vi "Unregister and Destroy Sessions.vi"(8 "error in (no error)":errorcluster) -> (0 "error out":errorcluster)   [LabVIEW 2020, in "NI-DCPower Source DC Voltage.lvlib"]
uses:
  NI-DCPower Source DC Voltage.lvlib
  <vilib>/MeasurementLink/MeasurementLink Discovery Client/RPC Messages/ni_measurementlink_discovery_v1_ResolveServiceRequest.ctl
  <vilib>/MeasurementLink/MeasurementLink Session Management Client/RPC Messages/ni_measurementlink_sessionmanagement_v1_ReserveAllRegisteredSessionsRequest.ctl
  <vilib>/MeasurementLink/MeasurementLink Session Management Client/MeasurementLink Session Management Client.lvlib
  <vilib>/MeasurementLink/MeasurementLink Discovery Client/MeasurementLink Discovery Client.lvlib
  <vilib>/MeasurementLink/MeasurementLink Measurement Server/MeasurementLink Measurement Server.lvlib
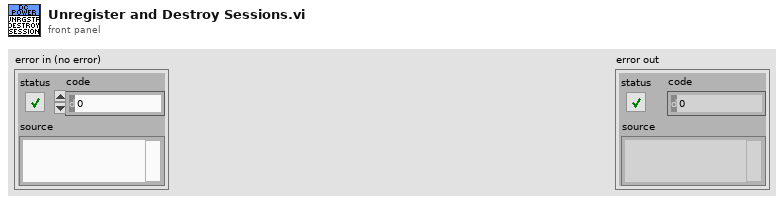
[diagram p1: front panel]
types:
  T1 = typedef "MeasurementLink Session Management Client.lvlib/ni_measurementlink_sessionmanagement_v1_ReserveAllRegisteredSessionsRequest.ctl" = cluster{"timeout_in_milliseconds":i32, "instrument_type_id":string}
  T2 = typedef "MeasurementLink Discovery Client.lvlib/ni_measurementlink_discovery_v1_ResolveServiceRequest.ctl" = cluster{"provided_interface":string, "service_class":string}
  T3 = typedef "grpc-lvsupport-release.lvlib/grpcId.ctl" = u64
  T4 = typedef "MeasurementLink Discovery Client.lvlib/ni_measurementlink_discovery_v1_ServiceLocation.ctl" = cluster{"location":string, "insecure_port":string, "ssl_authenticated_port":string}
  T5 = typedef "MeasurementLink Session Management Client.lvlib/ni_measurementlink_sessionmanagement_v1_ReserveAllRegisteredSessionsResponse.ctl" = cluster{"sessions":T6[]}
  T6 = typedef "MeasurementLink Session Management Client.lvlib/ni_measurementlink_sessionmanagement_v1_SessionInformation.ctl" = cluster{"session":T7, "resource_name":string, "channel_list":string, "instrument_type_id":string, "session_exists":bool, "channel_mappings":T8[]}
  T7 = typedef "MeasurementLink Session Management Client.lvlib/nidevice_grpc_Session.ctl" = cluster{"name":string}
  T8 = typedef "MeasurementLink Session Management Client.lvlib/ni_measurementlink_sessionmanagement_v1_ChannelMapping.ctl" = cluster{"pin_or_relay_name":string, "site":i32, "channel":string}
  T9 = cluster{"session Name":string, "address (localhost)":string, "port (31763)":i32}
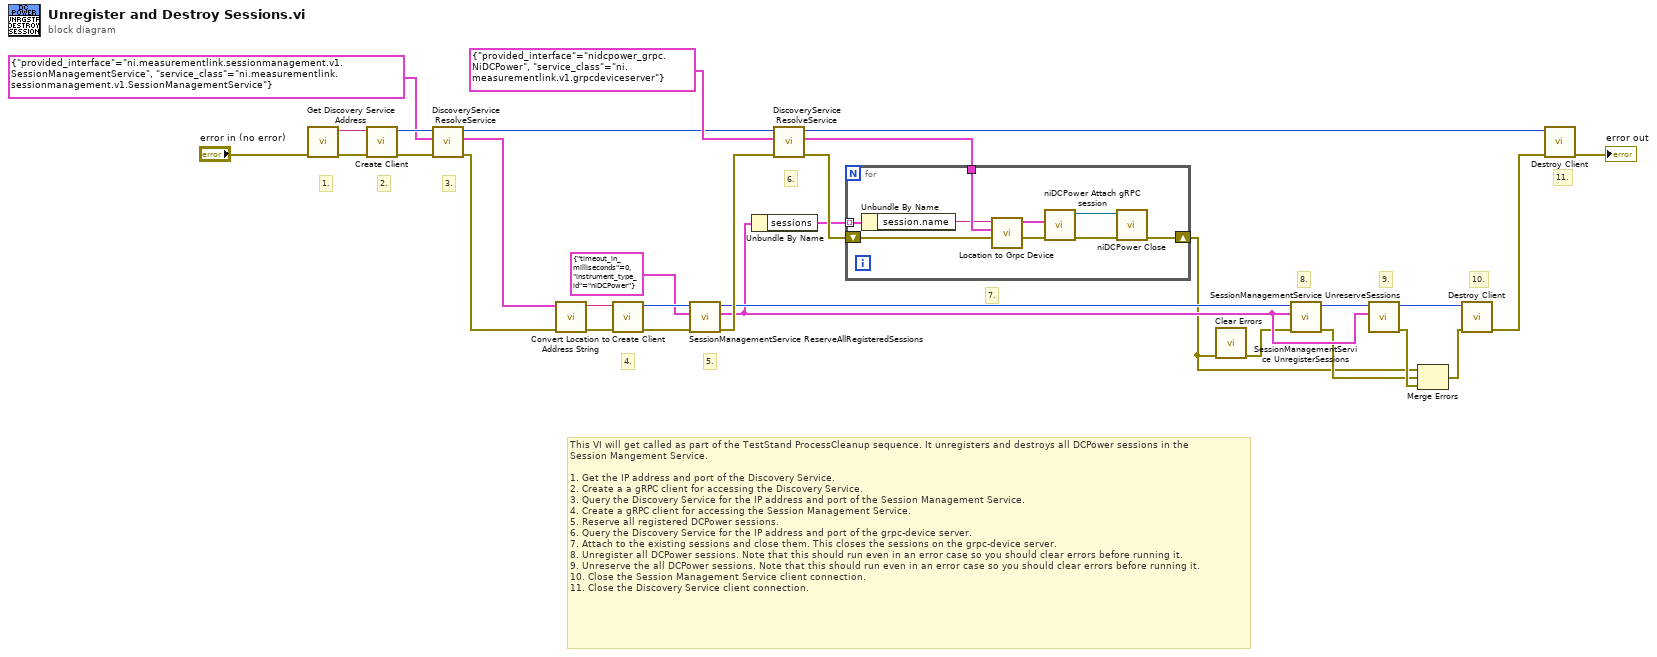
[diagram p0: block diagram]
diagram:
  # "11."
  # "10."
  # "9."
  # "8."
  # "7."
  # "6."
  # "5."
  # "4."
  # "3."
  # "2."
  # "1."
  # "This VI will get called as part of the TestStand ProcessCleanup sequence. It unregisters and destroys all DCPower sessions in the\nSession Mangement Service.\n\n1. Get the IP address and port of the Discovery Service.\n2. Create a a gRPC client for accessing the Discovery Service.\n3. Query the Discovery Service for the IP address and port of the Session Management Service.\n4. Create a gRPC client for accessing the Session Management Service.\n5. Reserve all registered DCPower sessions. \n6. Query the Discovery Service for the IP address and port of the grpc-device server.\n7. Attach to the existing sessions and close them. This closes the sessions on the grpc-device server.\n8. Unregister all DCPower sessions. Note that this should run even in an error case so you should clear errors before running it.\n9. Unreserve the all DCPower sessions. Note that this should run even in an error case so you should clear errors before running it.\n10. Close the Session Management Service client connection.\n11. Close the Discovery Service client connection."
  n1 = call <vilib>:"Get Discovery Service Address.vi"("error in"="error in (no error)") -> ("error out"=w12:errorcluster, "address"=w11:string)  [unwired: 9 in]
  n2 = call <vilib>:"Create Client.vi"("error in"=w12, "address"=w11) -> ("error out"=w29:errorcluster, "gRPC ID Out"=w30:T3)  [unwired: 8 in]
  n3 = call <vilib>:"DiscoveryService ResolveService.vi"("error in"=w29, "Request Data"=T2 {"provided_interface"="ni.measurementlink.sessionmanagement.v1.SessionManagementService", "service_class"="ni.measurementlink.sessionmanagement.v1.SessionManagementService"}, "gRPC ID"=w30) -> ("error out"=w9:errorcluster, "Response Data"=w8:T4, "gRPC ID out"=w23:T3)  [unwired: 6 in]
  n4 = call "Convert Location to Address String.vi"("Response Data"=w8) -> ("String"=w7:string)  [unwired: 10 in]
  n5 = call <vilib>:"Create Client.vi"("error in"=w9, "address"=w7) -> ("error out"=w19:errorcluster, "gRPC ID Out"=w18:T3)  [unwired: 8 in]
  n6 = call <vilib>:"SessionManagementService ReserveAllRegisteredSessions.vi"("error in"=w19, "Request Data"=T1 {"timeout_in_milliseconds"=0, "instrument_type_id"="niDCPower"}, "gRPC ID"=w18) -> ("error out"=w16:errorcluster, "Response Data"=w6:T5, "gRPC ID out"=w15:T3)  [unwired: 6 in]
  n7 = Unbundle By Name(w6) -> ("sessions"=w13:T6[])
  n8 = call <vilib>:"DiscoveryService ResolveService.vi"("error in"=w16, "Request Data"=T2 {"provided_interface"="nidcpower_grpc.NiDCPower", "service_class"="ni.measurementlink.v1.grpcdeviceserver"}, "gRPC ID"=w23) -> ("error out"=w21:errorcluster, "Response Data"=w20:T4, "gRPC ID out"=w22:T3)  [unwired: 6 in]
  n9 = for {
    tunnel: w13 -> [w33] mode=indexing
    shift-right: [w36] -> w2
    shift-left: w21 -> [w31]
    tunnel: w20 -> [w34]
    n10 = Unbundle By Name(w33) -> ("session.name"=w32:string)
    n11 = call "Location to Grpc Device.vi"("Grpc Device Location"=w34, "Session Name"=w32) -> ("NI gRPC Device Server Out"=w35:T9)  [unwired: 9 in]
    n12 = call <instrlib>:"niDCPower Attach gRPC session.vi"("error in (no error)"=w31, "NI gRPC Device Server"=w35) -> ("error out"=w38:errorcluster, "instrument handle out"=w37:refnum<k15>)  [unwired: 8 in]
    n13 = call <instrlib>:"niDCPower Close.vi"("error in (no error)"=w38, "instrument handle"=w37) -> ("error out"=w36:errorcluster)  [unwired: 9 in]
  }
  n14 = call <vilib>:"Clear Errors.vi"("error in (no error)"=w2) -> ("error out"=w1:errorcluster)  [unwired: 5 in, 1 out]
  n15 = call <vilib>:"SessionManagementService UnregisterSessions.vi"("error in"=w1, "Request Data"=w6, "gRPC ID"=w15) -> ("error out"=w3:errorcluster, "gRPC ID out"=w14:T3)  [unwired: 6 in, 1 out]
  n16 = call <vilib>:"SessionManagementService UnreserveSessions.vi"("Request Data"=w6, "gRPC ID"=w14) -> ("error out"=w5:errorcluster, "gRPC ID out"=w24:T3)  [unwired: 7 in, 1 out]
  n17 = Merge Errors(w2, w3, w5) -> (w4:errorcluster)
  n18 = call <vilib>:"Destroy Client.vi"("error in"=w4, "gRPC ID"=w24) -> ("error out"=w28:errorcluster)  [unwired: 9 in]
  n19 = call <vilib>:"Destroy Client.vi"("error in"=w28, "gRPC ID"=w22) -> ("error out"=→"error out":errorcluster)  [unwired: 9 in]
